vi "QualisysInstruction.vi"() -> ()   [LabVIEW 2017]
panel:
  in  "CommandeQualisys":string
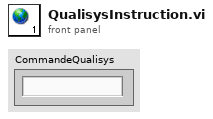
[diagram p1: front panel]
diagram:
